vi "Read.vi"(8 "error in (no error)":errorcluster, 9 "timeout in ms (60 sec)":i32=60000, 11 "Future in":refnum<class "Future.lvclass">) -> (0 "error out":errorcluster, 1 "Result Error":errorcluster, 2 "Result Value":variant, 4 "Timed Out":bool)   [LabVIEW 2017, in "Futures.lvlib" / "Future.lvclass"]
doc: "Read the result of the future.\n\nIf the future is resolved then the future becomes invalidated and cannot be read again.\n\nIf the future times out then you can attempt another read."
uses:
  Future.lvclass
  Future.lvclass/Future.ctl
  <vilib>/Utility/error.llb/Error Cluster From Error Code.vi
  Result/Result.lvclass
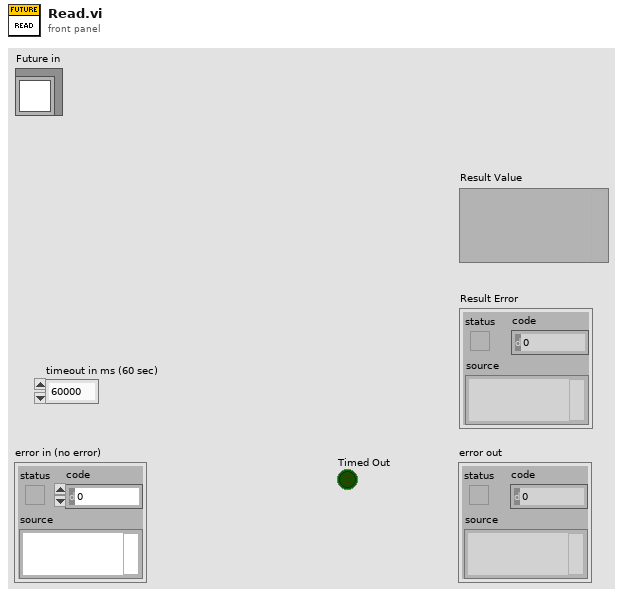
[diagram p1: front panel]
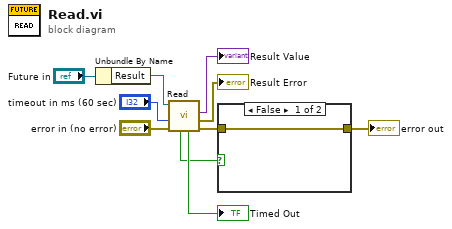
[diagram p0: block diagram]
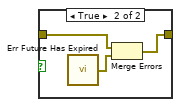
[diagram p2: hidden frame]
diagram:
  n1 = Unbundle By Name("Future in") -> ("Result"=w4:refnum<class "Result.lvclass">)
  n2 = call "Read.vi"("error in (no error)"="error in (no error)", "timeout in ms (60 sec)"="timeout in ms (60 sec)", "Result in"=w4) -> ("error out"=w2:errorcluster, "Result Error"=→"Result Error":errorcluster, "Result Value"=→"Result Value":variant, "Timed Out?"=→"Timed Out":bool, "Future Has Expired"=w3:bool)  [unwired: 4 in]
  n3 = case shown="False" w3 {
    tunnel: w2 -> [w11 w13]
    tunnel: [w11 w14] -> w1
    frame False {
    }
    frame True {
      n4 = call "Err Future Has Expired.vi"() -> ("Future Expired"=w12:errorcluster)
      n5 = Merge Errors(w13, w12) -> (w14:errorcluster)
    }
  }
  "error out" <- w1
